vi "Plugin.Initialize.vi"(8 "error in (no error)":errorcluster, 10 "Transfers":refnum<class "DSF.Engine.Transfer.lvclass">[](array[class]), 11 "Plugin in":refnum<class "Plugin.lvclass">) -> (0 "error out":errorcluster, 3 "Plugin out":refnum<class "Plugin.lvclass">)   [LabVIEW 2016, in "Plugin.lvclass"]
uses:
  Plugin.lvclass
  Source/Engine/Classes/Transfer/DSF.Engine.Transfer.lvclass
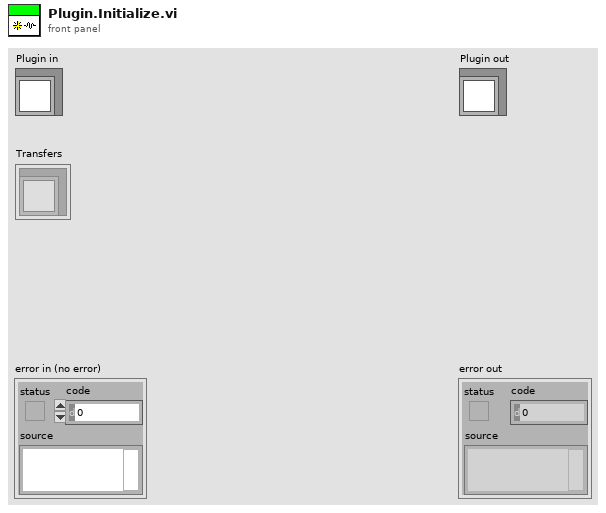
[diagram p1: front panel]
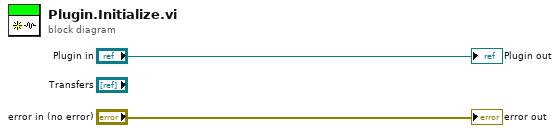
[diagram p0: block diagram]
diagram:
  "error out" <- "error in (no error)"
  "Plugin out" <- "Plugin in"
